vi "Get DAQ AI ScanArray Data.vi"(0 "DAQ":refnum<class "DAQ.lvclass">, 5 "DataName":string="AIScanArray", 11 "error in (no error)":errorcluster) -> (4 "DAQ":refnum<class "DAQ.lvclass">, 6 "AI ScanArray":dbl[](array[numeric]), 8 "Timestamp (DBL)":dbl, 10 "Time Stamp":timestamp, 15 "error out":errorcluster)   [LabVIEW 2022 SP3, in "DAQ.lvclass"]
doc: "Developed by Kevin Thompson\nkevin@thompsonengineering.net\n\nCopyright 2018-2020\nThompson Engineering, LLC\nThis public method retrieves the scanned analog inputs (AI) as an array, in the order of the AI IOName TD enum."
uses:
  DAQ.lvclass
  Process/ProcessSupport/TD DaqThread--enum.ctl
  DAQ.lvclass/DAQ.ctl
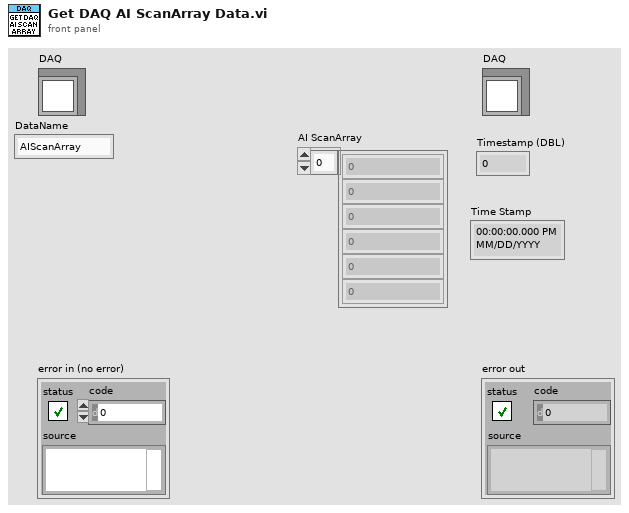
[diagram p1: front panel]
types:
  T1 = typedef "DAQ.lvclass/TD DaqThread--enum.ctl" = enum16{"AI", "DI"}
  T2 = typedef "TD Dynamic CVT DVR--ref.ctl" = refnum<data-value>
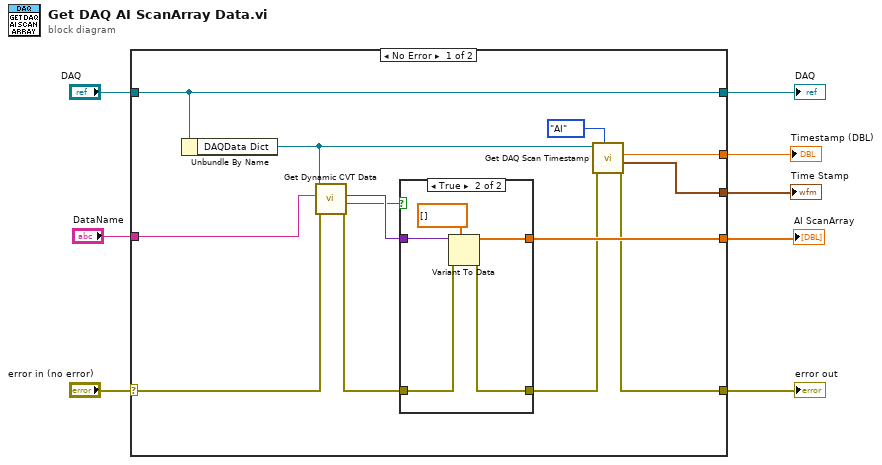
[diagram p0: block diagram]
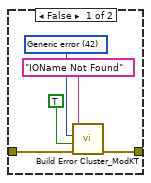
[diagram p2: hidden frame]
diagram:
  n1 = case shown="No Error" "error in (no error)" {
    selector: "error in (no error)" -> [w16 w33]
    tunnel: [w14 w33] -> w7
    tunnel: [w21 w32] -> w5
    tunnel: "DAQ" -> [w21 w32]
    tunnel: [w17 _] -> w4
    tunnel: [w11 _] -> w3
    tunnel: [w10 _] -> w2
    tunnel: "DataName" -> [w9 _]
    frame No Error {
      n2 = Unbundle By Name(w21) -> ("DAQData Dict"=w15:T2)
      n3 = call <vilib>:"Get Dynamic CVT Data.vi"("error in (no error)"=w16, "DataName"=w9, "dCVT DVR"=w15) -> ("error out"=w20:errorcluster, "found"=w18:bool, "value"=w19:variant)  [unwired: 5 in, 1 out]
      n4 = case shown="True" w18 {
        tunnel: w20 -> [w23 w31]
        tunnel: [w22 w30] -> w13
        tunnel: w19 -> [_ w29]
        tunnel: [_ w28] -> w17
        frame False {
          w25 = 42 items=["No error", "Argument error", "Memory is full", "Out of zone", "End of file", "File already open", "Generic file I/O error", "File not found", "File permission error", "Disk is full", "Duplicate path", "Too many files open", "System feature not enabled", "Resource file not found", "Cannot add resource", "Resource not found", "Image not found", "Image memory error", "Pen does not exist", "Config type invalid", "Config token not found", "Config parse error", "Config memory error", "Bad external code format", "Bad external code offset", "External code not present", "Null window", "Destroy window error", "Null menu", "Print aborted", "Bad print record", "Print driver error", "Windows error during printing", "Memory error during printing", "Print dialog error", "Generic print error", "Invalid device refnum", "Device not found", "Device parameter error", "Device unit error", "Cannot open device", "Device call aborted", "Generic error", "Cancelled by user", "Object ID too low", "Object ID too high", "Object not in heap", "Unknown heap", "Unknown object (invalid DefProc)", "Unknown object (DefProc not in table)", "Message out of range", "Invalid (null) method", "Unknown message", "Manager call not supported", "Bad address", "Network operation in progress", "Network operation timed out", "Connection is busy", "Network attribute not supported", "Network error", "Address in use", "System out of memory", "Connection aborted", "Connection refused", "Not connected", "Already connected", "Connection closed", "Initialization error (interapplication manager)", "Bad occurrence", "Wait on unbound occurrence handler", "Occurrence queue overflow", "Datalog type conflict", "Unused", "Unrecognized type (interapplication manager)", "Memory corrupt", "Failed to make temporary DLL", "Old CIN version", "Drag socket not found", "Failed to load drop-object", "Failed to register OLE object", "Failed to release OLE object", "Format specifier type mismatch", "Unknown format specifier", "Too few format specifiers", "Too many format specifiers", "Scan failed", "Newer CIN version", "Error converting to variant", "Runtime menu error", "Password tampered", "Variant attribute not found", "Incompatible variant data type", "Event data is not available", "Event Store is not present", "Occurrence is not found", "Event Queue is not created", "Event info is not available", "Refnum passed is NULL", "Error retrieving Class GUID", "Error retrieving CoClass GUID", "Error retrieving TypeLib GUID.", "Bad built application magic bytes.", "Specific driver is different from the specific driver associated with the Logical Name.", "There is no session opened to the class driver.", "Max Error", "MAX - Error with config objects", "MAX - Error loading configuration", "MAX - Group not supported"]
          n5 = call <vilib>:"Build Error Cluster_ModKT .vi"("Prepend String (\"\")"="IOName Not Found" ("Prepend String (\"\")"), "code"=w25, "error? (F)"=TRUE, "error in (no error)"=w23) -> ("error out"=w22:errorcluster)  [unwired: 3 in, 1 out]
        }
        frame True {
          n6 = Variant To Data(error in=w31, type=dbl[] [], Variant=w29) -> (data=w28:dbl[], error out=w30:errorcluster)
        }
      }
      n7 = call "Get DAQ Scan Timestamp.vi"("Daq Thread"=TD_DaqThread--enum."AI", "error in (no error)"=w13, "DaqData dCVT"=w15) -> ("error out"=w14:errorcluster, "Time Stamp"=w10:timestamp, "Timestamp (DBL)"=w11:dbl)  [unwired: 5 in, 1 out]
    }
    frame Error {
    }
  }
  "error out" <- w7
  "DAQ" <- w5
  "AI ScanArray" <- w4
  "Timestamp (DBL)" <- w3
  "Time Stamp" <- w2
